vi "Shooter Button SUBVI.vi"   [LabVIEW 2011]
types:
  T1 = cluster{"Digital Input [1-16][0]":bool, "Digital Input [1-16][1]":bool, "Digital Input [1-16][2]":bool, "Digital Input [1-16][3]":bool, "Digital Input [1-16][4]":bool, "Digital Input [1-16][5]":bool, "Digital Input [1-16][6]":bool, "Digital Input [1-16][7]":bool, "Digital Input [1-16][8]":bool, "Digital Input [1-16][9]":bool, "Digital Input [1-16][10]":bool, "Digital Input [1-16][11]":bool, "Digital Input [1-16][12]":bool, "Digital Input [1-16][13]":bool, "Digital Input [1-16][14]":bool, "Digital Input [1-16][15]":bool}
  T2 = typedef "WPI_JoystickDevRef.ctl" = cluster{"Device":T3}
  T3 = typedef "WPI_JoystickDeviceEnum.ctl" = enum16{"USB 1", "USB 2", "USB 3", "USB 4", "Kinect 1", "Kinect 2"}
  T4 = typedef "WPI_JoystickButtonState.ctl" = cluster{"Button 1":bool, "Button 2":bool, "Button 3":bool, "Button 4":bool, "Button 5":bool, "Button 6":bool, "Button 7":bool, "Button 8":bool, "Button 9":bool, "Button 10":bool, "Button 11":bool, "Button 12":bool}
  T5 = cluster{"axis 1 (x)":dbl, "axis 2 (y)":dbl, "axis 3 (throttle)":dbl, "axis 4":dbl, "axis 5":dbl, "axis 6":dbl}
  T6 = typedef "WPI_DigitalInputDevRef.ctl" = cluster{"DevStatus":errorcluster, "DIO Channel":T7, "Digital Module":T8}
  T7 = typedef "FPGA_DIOChannel.ctl" = enum8{"DIO 1", "DIO 2", "DIO 3", "DIO 4", "DIO 5", "DIO 6", "DIO 7", "DIO 8", "DIO 9", "DIO 10", "DIO 11", "DIO 12", "DIO 13", "DIO 14", "Invalid"}
  T8 = typedef "FPGA_TypedefDigitalModule.ctl" = enum16{"Digital Module 1", "Digital Module 2"}
  T9 = typedef "WPI_MotorControlDeviceRef.ctl" = cluster{"DeviceStatus":errorcluster, "Type":enum16{"PWM", "CAN"}, "PWM":cluster{"Digital Module":T8, "PWM Channel":T10, "DeadBand":T11}, "CAN":cluster{"Device Number":u8, "Control Mode":T12, "Semaphore":T13, "Max Vout":dbl}, "Invert":bool, "TransformRef":T14, "InvTransformRef":T14}
  T10 = typedef "FPGA_DIOPWMChannel.ctl" = enum8{"PWM 1", "PWM 2", "PWM 3", "PWM 4", "PWM 5", "PWM 6", "PWM 7", "PWM 8", "PWM 9", "PWM 10", "Invalid"}
  T11 = typedef "WPI_PWMDeadband.ctl" = cluster{"Name":string, "maxPositivePwm":i32, "minPositivePwm":i32, "centerPwm":i32, "maxNegativePwm":i32, "minNegativePwm":i32, "angularRange":u16}
  T12 = typedef "WPI_CANJaguar_ControlMode.ctl" = enum8{"Percent VBus", "Current", "Speed", "Position", "Voltage"}
  T13 = typedef "Semaphore RefNum" = refnum<k1>
  T14 = typedef "WPI_PWMTransform_ConPane.ctl" = refnum<vi>
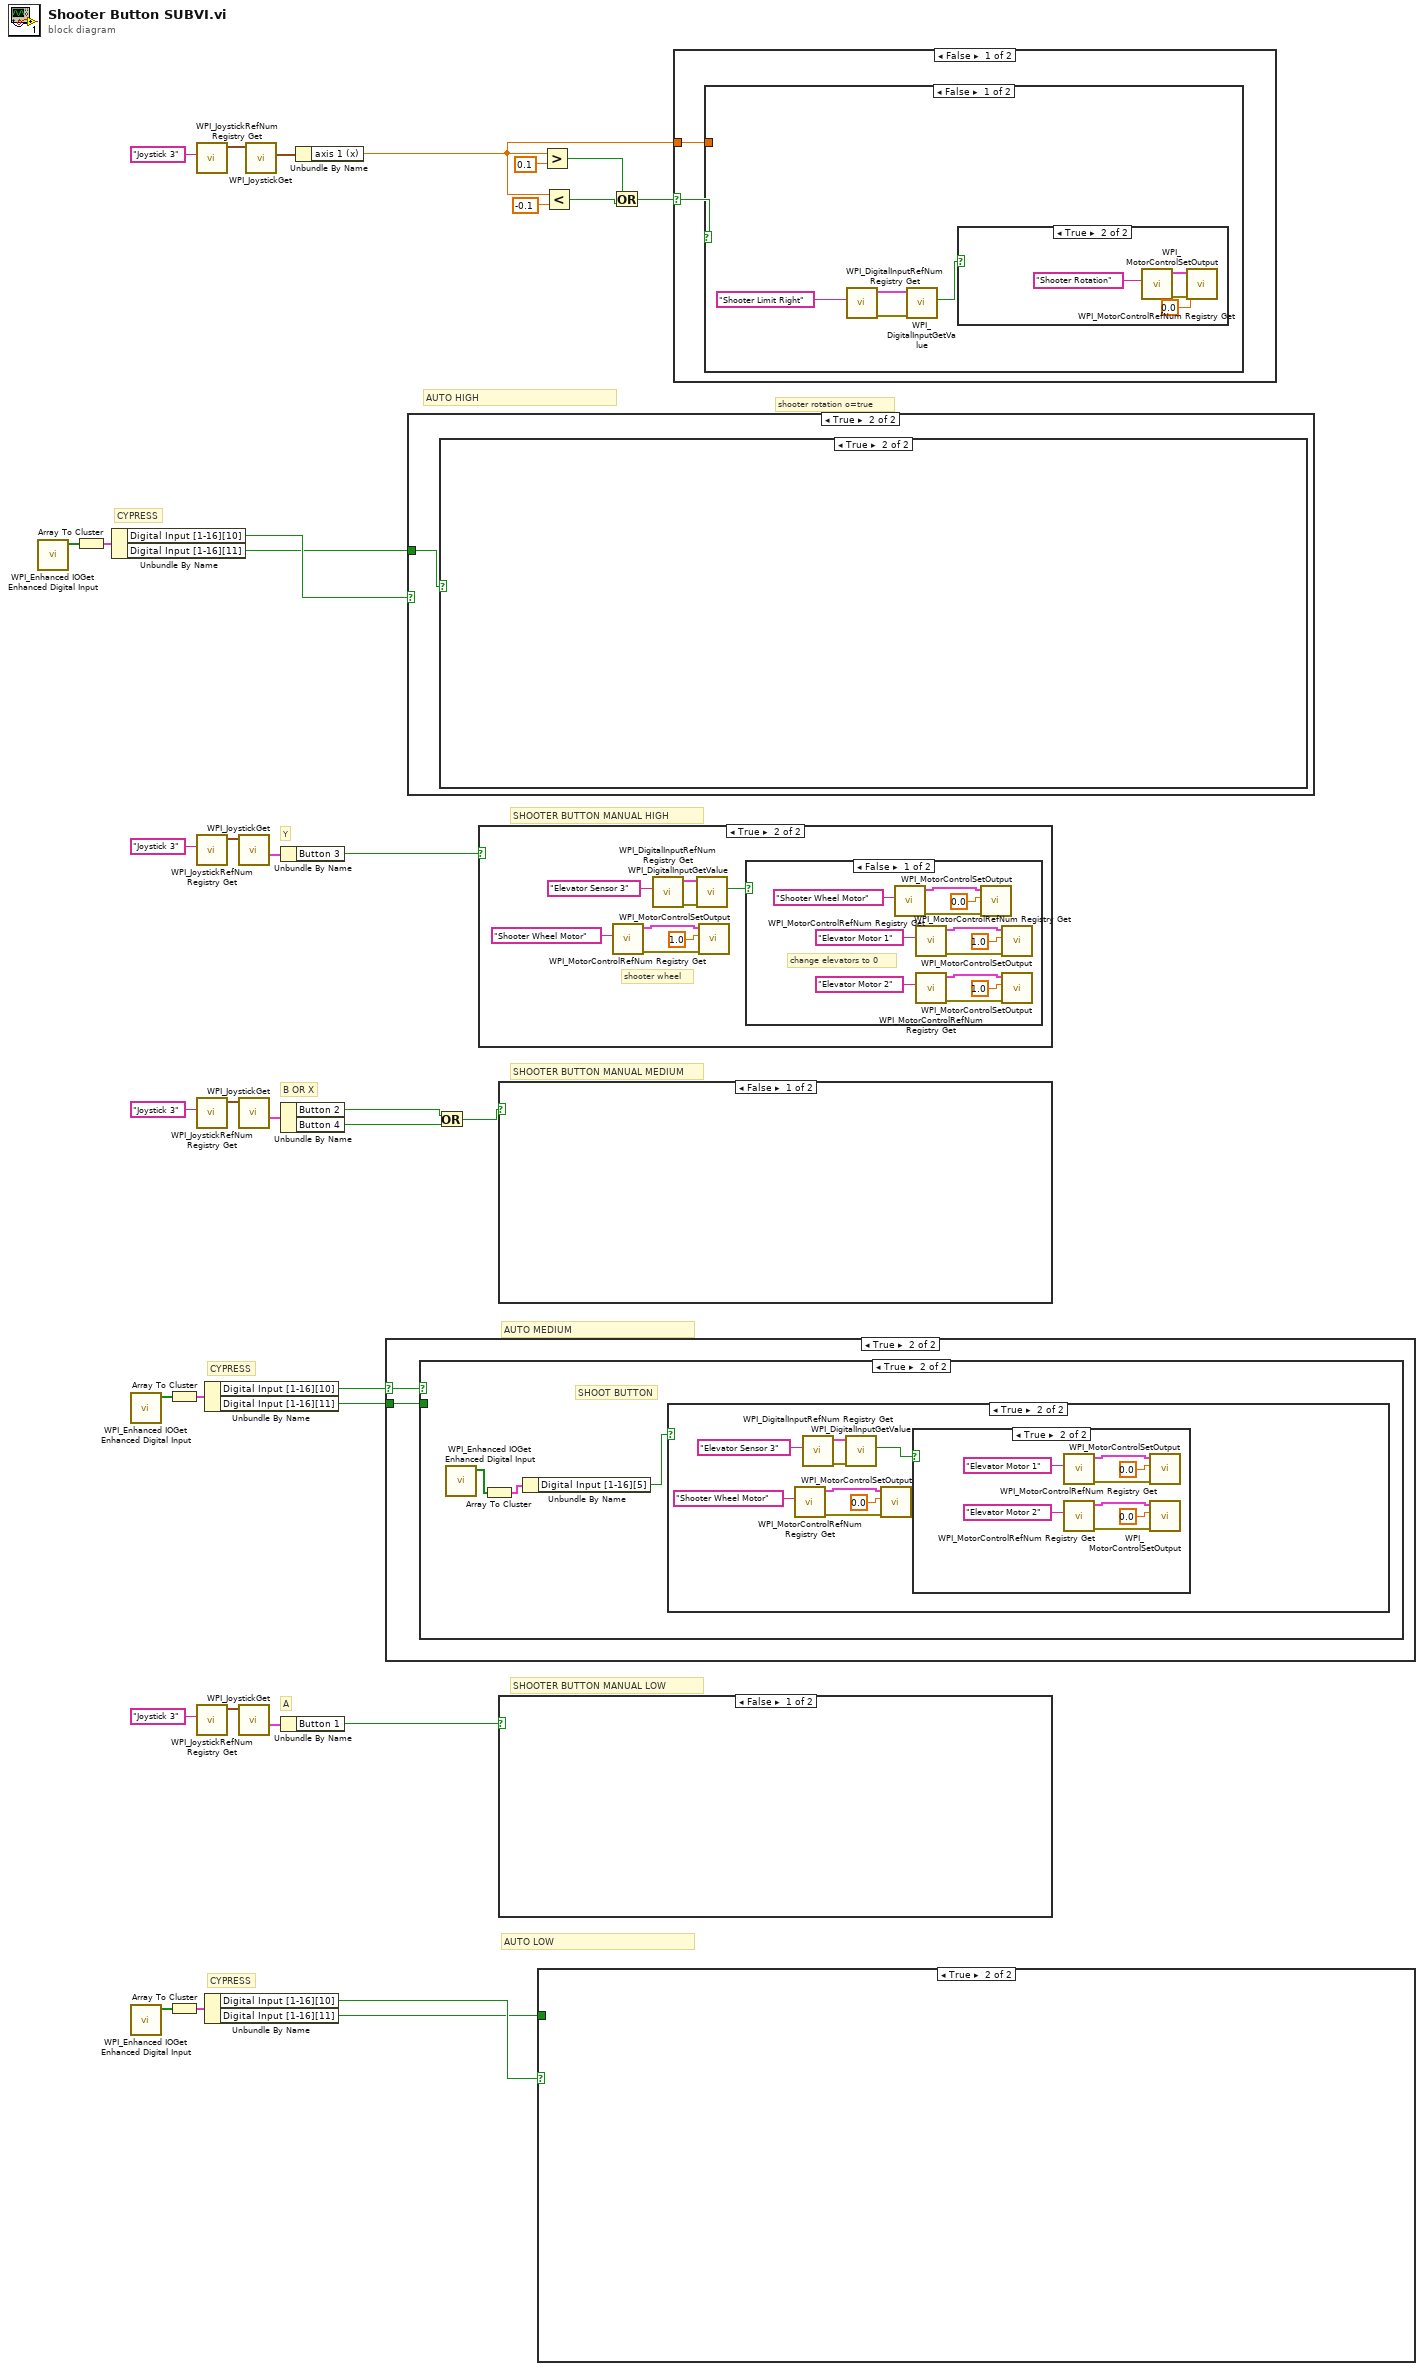
[diagram p0: block diagram]
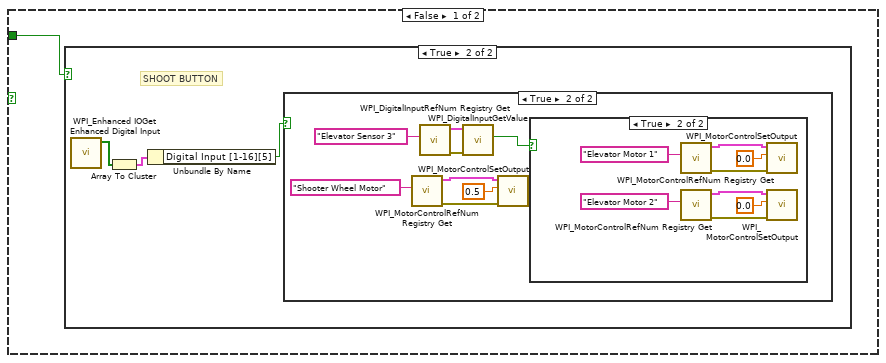
[diagram p2: hidden frame]
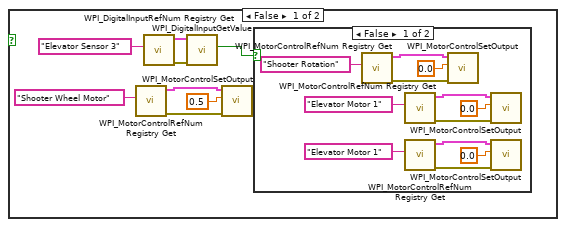
[diagram p4: hidden frame]
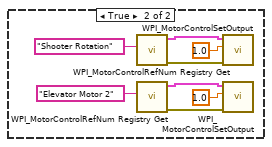
[diagram p5: hidden frame]
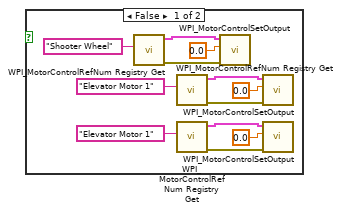
[diagram p6: hidden frame]
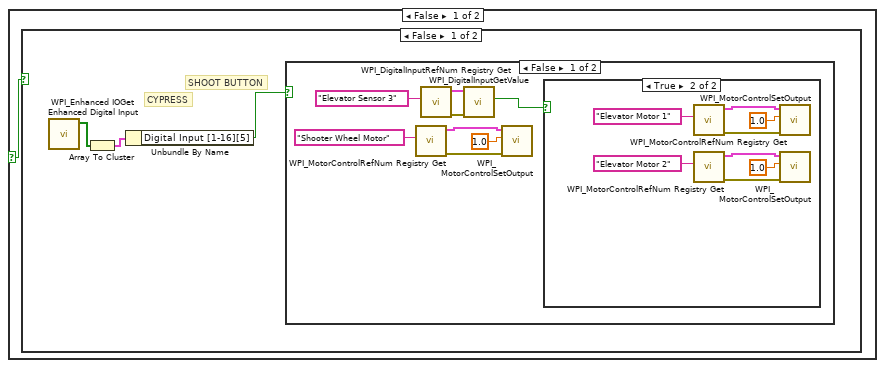
[diagram p8: hidden frame]
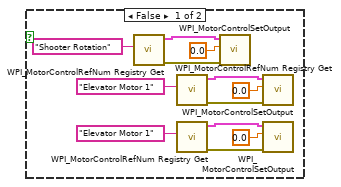
[diagram p9: hidden frame]
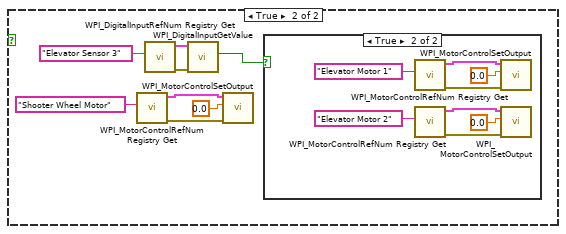
[diagram p10: hidden frame]
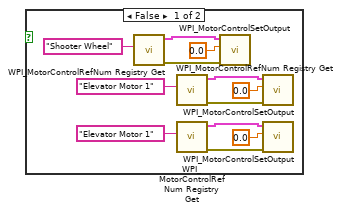
[diagram p11: hidden frame]
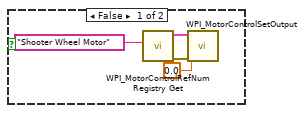
[diagram p13: hidden frame]
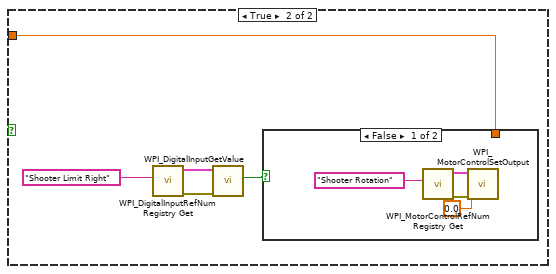
[diagram p14: hidden frame]
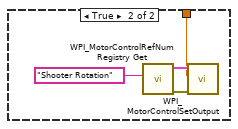
[diagram p15: hidden frame]
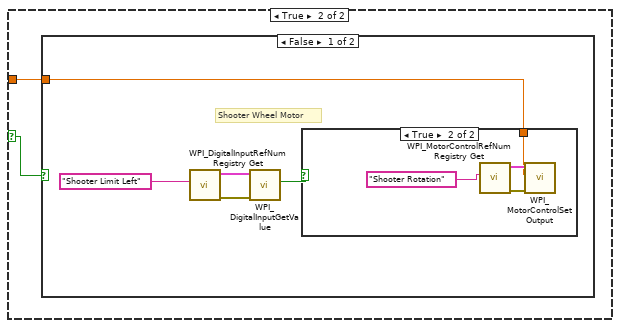
[diagram p16: hidden frame]
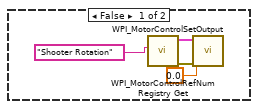
[diagram p17: hidden frame]
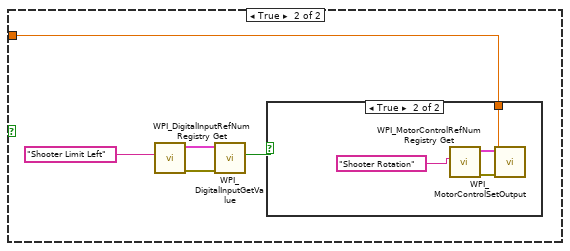
[diagram p18: hidden frame]
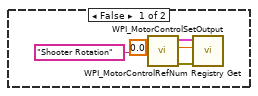
[diagram p19: hidden frame]
diagram:
  # "shooter rotation o=true"
  # "CYPRESS"
  # "CYPRESS"
  # "AUTO LOW"
  # "AUTO MEDIUM"
  # "A"
  # "B OR X"
  # "Y"
  # "SHOOTER BUTTON MANUAL LOW"
  # "SHOOTER BUTTON MANUAL MEDIUM"
  # "SHOOTER BUTTON MANUAL HIGH"
  # "CYPRESS"
  # "AUTO HIGH"
  n1 = call <vilib>:"WPI_Enhanced IOGet Enhanced Digital Input.vi"() -> ("Digital Input [1-16]"=w24:bool[])  [unwired: 10 in, 1 out]
  n2 = Array To Cluster(array=w24) -> (cluster=w23:T1)
  n3 = Unbundle By Name(w23) -> ("Digital Input [1-16][10]"=w8:bool, "Digital Input [1-16][11]"=w7:bool)
  n4 = call <vilib>:"WPI_Enhanced IOGet Enhanced Digital Input.vi"() -> ("Digital Input [1-16]"=w22:bool[])  [unwired: 10 in, 1 out]
  n5 = call <vilib>:"WPI_Enhanced IOGet Enhanced Digital Input.vi"() -> ("Digital Input [1-16]"=w20:bool[])  [unwired: 10 in, 1 out]
  n6 = Array To Cluster(array=w22) -> (cluster=w21:T1)
  n7 = Array To Cluster(array=w20) -> (cluster=w19:T1)
  n8 = call <vilib>:"WPI_JoystickRefNum Registry Get.vi"("refnum name"="Joystick 3") -> ("JoystickDevRef"=w17:T2)  [unwired: 9 in, 1 out]
  n9 = call <vilib>:"WPI_JoystickRefNum Registry Get.vi"("refnum name"="Joystick 3") -> ("JoystickDevRef"=w35:T2)  [unwired: 9 in, 1 out]
  n10 = call <vilib>:"WPI_JoystickRefNum Registry Get.vi"("refnum name"="Joystick 3") -> ("JoystickDevRef"=w32:T2)  [unwired: 9 in, 1 out]
  n11 = call <vilib>:"WPI_JoystickRefNum Registry Get.vi"("refnum name"="Joystick 3") -> ("JoystickDevRef"=w29:T2)  [unwired: 9 in, 1 out]
  n12 = Unbundle By Name(w21) -> ("Digital Input [1-16][10]"=w18:bool, "Digital Input [1-16][11]"=w6:bool)
  n13 = Unbundle By Name(w19) -> ("Digital Input [1-16][10]"=w5:bool, "Digital Input [1-16][11]"=w4:bool)
  n14 = call <vilib>:"WPI_JoystickGet.vi"("JoystickDevRef"=w35) -> ("Buttons"=w34:T4)  [unwired: 4 in, 2 out]
  n15 = call <vilib>:"WPI_JoystickGet.vi"("JoystickDevRef"=w32) -> ("Buttons"=w30:T4)  [unwired: 4 in, 2 out]
  n16 = call <vilib>:"WPI_JoystickGet.vi"("JoystickDevRef"=w29) -> ("Buttons"=w27:T4)  [unwired: 4 in, 2 out]
  n17 = call <vilib>:"WPI_JoystickGet.vi"("JoystickDevRef"=w17) -> ("Axes"=w15:T5)  [unwired: 4 in, 2 out]
  n18 = Unbundle By Name(w34) -> ("Button 3"=w33:bool)
  n19 = Unbundle By Name(w30) -> ("Button 2"=w3:bool, "Button 4"=w2:bool)
  n20 = Unbundle By Name(w27) -> ("Button 1"=w26:bool)
  n21 = Unbundle By Name(w15) -> ("axis 1 (x)"=w11:dbl)
  n22 = case shown="True" w18 {
    selector: w18 -> [_ w37]
    tunnel: w6 -> [_ w36]
    frame False {
    }
    frame True {
      n23 = case shown="True" w37 {
        tunnel: w36 -> [_ _]
        frame False {
        }
        frame True {
          # "SHOOT BUTTON"
          n24 = call <vilib>:"WPI_Enhanced IOGet Enhanced Digital Input.vi"() -> ("Digital Input [1-16]"=w40:bool[])  [unwired: 10 in, 1 out]
          n25 = Array To Cluster(array=w40) -> (cluster=w39:T1)
          n26 = Unbundle By Name(w39) -> ("Digital Input [1-16][5]"=w38:bool)
          n27 = case shown="True" w38 {
            frame False {
              n28 = call <vilib>:"WPI_DigitalInputRefNum Registry Get.vi"("refnum name"="Elevator Sensor 3") -> ("error out"=w47:errorcluster, "DigitalInputDevRef"=w46:T6)  [unwired: 9 in]
              n29 = call <vilib>:"WPI_MotorControlRefNum Registry Get.vi"("refnum name"="Shooter Wheel Motor") -> ("error out"=w44:errorcluster, "MotorControlDevRef"=w43:T9)  [unwired: 9 in]
              n30 = call <vilib>:"WPI_DigitalInputGetValue.vi"("error in (no error)"=w47, "DigitalInputDevRef"=w46) -> ("Value"=w45:bool)  [unwired: 7 in, 2 out]
              n31 = call <vilib>:"WPI_MotorControlSetOutput.vi"("error in (no error)"=w44, "Output"=0.75, "MotorControlDevRef"=w43) -> ()  [unwired: 7 in, 2 out]
              n32 = case shown="True" w45 {
                frame False {
                  n33 = call <vilib>:"WPI_MotorControlRefNum Registry Get.vi"("refnum name"="Shooter Rotation") -> ("error out"=w52:errorcluster, "MotorControlDevRef"=w51:T9)  [unwired: 9 in]
                  n34 = call <vilib>:"WPI_MotorControlRefNum Registry Get.vi"("refnum name"="Elevator Motor 1") -> ("error out"=w56:errorcluster, "MotorControlDevRef"=w55:T9)  [unwired: 9 in]
                  n35 = call <vilib>:"WPI_MotorControlRefNum Registry Get.vi"("refnum name"="Elevator Motor 1") -> ("error out"=w60:errorcluster, "MotorControlDevRef"=w59:T9)  [unwired: 9 in]
                  n36 = call <vilib>:"WPI_MotorControlSetOutput.vi"("error in (no error)"=w52, "Output"=0.0, "MotorControlDevRef"=w51) -> ()  [unwired: 7 in, 2 out]
                  n37 = call <vilib>:"WPI_MotorControlSetOutput.vi"("error in (no error)"=w56, "Output"=0.0, "MotorControlDevRef"=w55) -> ()  [unwired: 7 in, 2 out]
                  n38 = call <vilib>:"WPI_MotorControlSetOutput.vi"("error in (no error)"=w60, "Output"=0.0, "MotorControlDevRef"=w59) -> ()  [unwired: 7 in, 2 out]
                }
                frame True {
                  n39 = call <vilib>:"WPI_MotorControlRefNum Registry Get.vi"("refnum name"="Elevator Motor 1") -> ("error out"=w64:errorcluster, "MotorControlDevRef"=w63:T9)  [unwired: 9 in]
                  n40 = call <vilib>:"WPI_MotorControlRefNum Registry Get.vi"("refnum name"="Elevator Motor 2") -> ("error out"=w68:errorcluster, "MotorControlDevRef"=w67:T9)  [unwired: 9 in]
                  n41 = call <vilib>:"WPI_MotorControlSetOutput.vi"("error in (no error)"=w64, "Output"=1.0, "MotorControlDevRef"=w63) -> ()  [unwired: 7 in, 2 out]
                  n42 = call <vilib>:"WPI_MotorControlSetOutput.vi"("error in (no error)"=w68, "Output"=1.0, "MotorControlDevRef"=w67) -> ()  [unwired: 7 in, 2 out]
                }
              }
            }
            frame True {
              n43 = call <vilib>:"WPI_MotorControlRefNum Registry Get.vi"("refnum name"="Shooter Wheel Motor") -> ("error out"=w72:errorcluster, "MotorControlDevRef"=w71:T9)  [unwired: 9 in]
              n44 = call <vilib>:"WPI_DigitalInputRefNum Registry Get.vi"("refnum name"="Elevator Sensor 3") -> ("error out"=w75:errorcluster, "DigitalInputDevRef"=w74:T6)  [unwired: 9 in]
              n45 = call <vilib>:"WPI_DigitalInputGetValue.vi"("error in (no error)"=w75, "DigitalInputDevRef"=w74) -> ("Value"=w73:bool)  [unwired: 7 in, 2 out]
              n46 = call <vilib>:"WPI_MotorControlSetOutput.vi"("error in (no error)"=w72, "Output"=0.0, "MotorControlDevRef"=w71) -> ()  [unwired: 7 in, 2 out]
              n47 = case shown="True" w73 {
                frame False {
                  n48 = call <vilib>:"WPI_MotorControlRefNum Registry Get.vi"("refnum name"="Shooter Wheel") -> ("error out"=w80:errorcluster, "MotorControlDevRef"=w79:T9)  [unwired: 9 in]
                  n49 = call <vilib>:"WPI_MotorControlRefNum Registry Get.vi"("refnum name"="Elevator Motor 1") -> ("error out"=w84:errorcluster, "MotorControlDevRef"=w83:T9)  [unwired: 9 in]
                  n50 = call <vilib>:"WPI_MotorControlRefNum Registry Get.vi"("refnum name"="Elevator Motor 1") -> ("error out"=w88:errorcluster, "MotorControlDevRef"=w87:T9)  [unwired: 9 in]
                  n51 = call <vilib>:"WPI_MotorControlSetOutput.vi"("error in (no error)"=w80, "Output"=0.0, "MotorControlDevRef"=w79) -> ()  [unwired: 7 in, 2 out]
                  n52 = call <vilib>:"WPI_MotorControlSetOutput.vi"("error in (no error)"=w84, "Output"=0.0, "MotorControlDevRef"=w83) -> ()  [unwired: 7 in, 2 out]
                  n53 = call <vilib>:"WPI_MotorControlSetOutput.vi"("error in (no error)"=w88, "Output"=0.0, "MotorControlDevRef"=w87) -> ()  [unwired: 7 in, 2 out]
                }
                frame True {
                  n54 = call <vilib>:"WPI_MotorControlRefNum Registry Get.vi"("refnum name"="Elevator Motor 1") -> ("error out"=w92:errorcluster, "MotorControlDevRef"=w91:T9)  [unwired: 9 in]
                  n55 = call <vilib>:"WPI_MotorControlRefNum Registry Get.vi"("refnum name"="Elevator Motor 2") -> ("error out"=w96:errorcluster, "MotorControlDevRef"=w95:T9)  [unwired: 9 in]
                  n56 = call <vilib>:"WPI_MotorControlSetOutput.vi"("error in (no error)"=w92, "Output"=0.0, "MotorControlDevRef"=w91) -> ()  [unwired: 7 in, 2 out]
                  n57 = call <vilib>:"WPI_MotorControlSetOutput.vi"("error in (no error)"=w96, "Output"=0.0, "MotorControlDevRef"=w95) -> ()  [unwired: 7 in, 2 out]
                }
              }
            }
          }
        }
      }
    }
  }
  n58 = case shown="True" w8 {
    tunnel: w7 -> [_ w97]
    frame False {
    }
    frame True {
      n59 = case shown="True" w97 {
        selector: w97 -> [w98 _]
        frame False {
          n60 = case shown="False" w98 {
            frame False {
              # "CYPRESS"
              # "SHOOT BUTTON"
              n61 = call <vilib>:"WPI_Enhanced IOGet Enhanced Digital Input.vi"() -> ("Digital Input [1-16]"=w101:bool[])  [unwired: 10 in, 1 out]
              n62 = Array To Cluster(array=w101) -> (cluster=w100:T1)
              n63 = Unbundle By Name(w100) -> ("Digital Input [1-16][5]"=w99:bool)
              n64 = case shown="False" w99 {
                frame False {
                  n65 = call <vilib>:"WPI_MotorControlRefNum Registry Get.vi"("refnum name"="Shooter Wheel Motor") -> ("error out"=w105:errorcluster, "MotorControlDevRef"=w104:T9)  [unwired: 9 in]
                  n66 = call <vilib>:"WPI_DigitalInputRefNum Registry Get.vi"("refnum name"="Elevator Sensor 3") -> ("error out"=w108:errorcluster, "DigitalInputDevRef"=w107:T6)  [unwired: 9 in]
                  n67 = call <vilib>:"WPI_DigitalInputGetValue.vi"("error in (no error)"=w108, "DigitalInputDevRef"=w107) -> ("Value"=w106:bool)  [unwired: 7 in, 2 out]
                  n68 = call <vilib>:"WPI_MotorControlSetOutput.vi"("error in (no error)"=w105, "Output"=1.0, "MotorControlDevRef"=w104) -> ()  [unwired: 7 in, 2 out]
                  n69 = case shown="True" w106 {
                    frame False {
                      n70 = call <vilib>:"WPI_MotorControlRefNum Registry Get.vi"("refnum name"="Shooter Rotation") -> ("error out"=w113:errorcluster, "MotorControlDevRef"=w112:T9)  [unwired: 9 in]
                      n71 = call <vilib>:"WPI_MotorControlRefNum Registry Get.vi"("refnum name"="Elevator Motor 1") -> ("error out"=w117:errorcluster, "MotorControlDevRef"=w116:T9)  [unwired: 9 in]
                      n72 = call <vilib>:"WPI_MotorControlRefNum Registry Get.vi"("refnum name"="Elevator Motor 1") -> ("error out"=w121:errorcluster, "MotorControlDevRef"=w120:T9)  [unwired: 9 in]
                      n73 = call <vilib>:"WPI_MotorControlSetOutput.vi"("error in (no error)"=w113, "Output"=0.0, "MotorControlDevRef"=w112) -> ()  [unwired: 7 in, 2 out]
                      n74 = call <vilib>:"WPI_MotorControlSetOutput.vi"("error in (no error)"=w117, "Output"=0.0, "MotorControlDevRef"=w116) -> ()  [unwired: 7 in, 2 out]
                      n75 = call <vilib>:"WPI_MotorControlSetOutput.vi"("error in (no error)"=w121, "Output"=0.0, "MotorControlDevRef"=w120) -> ()  [unwired: 7 in, 2 out]
                    }
                    frame True {
                      n76 = call <vilib>:"WPI_MotorControlRefNum Registry Get.vi"("refnum name"="Elevator Motor 1") -> ("error out"=w125:errorcluster, "MotorControlDevRef"=w124:T9)  [unwired: 9 in]
                      n77 = call <vilib>:"WPI_MotorControlRefNum Registry Get.vi"("refnum name"="Elevator Motor 2") -> ("error out"=w129:errorcluster, "MotorControlDevRef"=w128:T9)  [unwired: 9 in]
                      n78 = call <vilib>:"WPI_MotorControlSetOutput.vi"("error in (no error)"=w125, "Output"=1.0, "MotorControlDevRef"=w124) -> ()  [unwired: 7 in, 2 out]
                      n79 = call <vilib>:"WPI_MotorControlSetOutput.vi"("error in (no error)"=w129, "Output"=1.0, "MotorControlDevRef"=w128) -> ()  [unwired: 7 in, 2 out]
                    }
                  }
                }
                frame True {
                  n80 = call <vilib>:"WPI_MotorControlRefNum Registry Get.vi"("refnum name"="Shooter Wheel Motor") -> ("error out"=w133:errorcluster, "MotorControlDevRef"=w132:T9)  [unwired: 9 in]
                  n81 = call <vilib>:"WPI_DigitalInputRefNum Registry Get.vi"("refnum name"="Elevator Sensor 3") -> ("error out"=w136:errorcluster, "DigitalInputDevRef"=w135:T6)  [unwired: 9 in]
                  n82 = call <vilib>:"WPI_DigitalInputGetValue.vi"("error in (no error)"=w136, "DigitalInputDevRef"=w135) -> ("Value"=w134:bool)  [unwired: 7 in, 2 out]
                  n83 = call <vilib>:"WPI_MotorControlSetOutput.vi"("error in (no error)"=w133, "Output"=0.0, "MotorControlDevRef"=w132) -> ()  [unwired: 7 in, 2 out]
                  n84 = case shown="True" w134 {
                    frame False {
                      n85 = call <vilib>:"WPI_MotorControlRefNum Registry Get.vi"("refnum name"="Shooter Wheel") -> ("error out"=w141:errorcluster, "MotorControlDevRef"=w140:T9)  [unwired: 9 in]
                      n86 = call <vilib>:"WPI_MotorControlRefNum Registry Get.vi"("refnum name"="Elevator Motor 1") -> ("error out"=w145:errorcluster, "MotorControlDevRef"=w144:T9)  [unwired: 9 in]
                      n87 = call <vilib>:"WPI_MotorControlRefNum Registry Get.vi"("refnum name"="Elevator Motor 1") -> ("error out"=w149:errorcluster, "MotorControlDevRef"=w148:T9)  [unwired: 9 in]
                      n88 = call <vilib>:"WPI_MotorControlSetOutput.vi"("error in (no error)"=w141, "Output"=0.0, "MotorControlDevRef"=w140) -> ()  [unwired: 7 in, 2 out]
                      n89 = call <vilib>:"WPI_MotorControlSetOutput.vi"("error in (no error)"=w145, "Output"=0.0, "MotorControlDevRef"=w144) -> ()  [unwired: 7 in, 2 out]
                      n90 = call <vilib>:"WPI_MotorControlSetOutput.vi"("error in (no error)"=w149, "Output"=0.0, "MotorControlDevRef"=w148) -> ()  [unwired: 7 in, 2 out]
                    }
                    frame True {
                      n91 = call <vilib>:"WPI_MotorControlRefNum Registry Get.vi"("refnum name"="Elevator Motor 1") -> ("error out"=w153:errorcluster, "MotorControlDevRef"=w152:T9)  [unwired: 9 in]
                      n92 = call <vilib>:"WPI_MotorControlRefNum Registry Get.vi"("refnum name"="Elevator Motor 2") -> ("error out"=w157:errorcluster, "MotorControlDevRef"=w156:T9)  [unwired: 9 in]
                      n93 = call <vilib>:"WPI_MotorControlSetOutput.vi"("error in (no error)"=w153, "Output"=0.0, "MotorControlDevRef"=w152) -> ()  [unwired: 7 in, 2 out]
                      n94 = call <vilib>:"WPI_MotorControlSetOutput.vi"("error in (no error)"=w157, "Output"=0.0, "MotorControlDevRef"=w156) -> ()  [unwired: 7 in, 2 out]
                    }
                  }
                }
              }
            }
            frame True {
            }
          }
        }
        frame True {
        }
      }
    }
  }
  n95 = Or(x=w3, y=w2) -> (x .or. y?=w1:bool)
  n96 = case shown="True" w33 {
    frame False {
    }
    frame True {
      # "shooter wheel"
      n97 = call <vilib>:"WPI_MotorControlRefNum Registry Get.vi"("refnum name"="Shooter Wheel Motor") -> ("error out"=w161:errorcluster, "MotorControlDevRef"=w160:T9)  [unwired: 9 in]
      n98 = call <vilib>:"WPI_DigitalInputRefNum Registry Get.vi"("refnum name"="Elevator Sensor 3") -> ("error out"=w164:errorcluster, "DigitalInputDevRef"=w163:T6)  [unwired: 9 in]
      n99 = call <vilib>:"WPI_DigitalInputGetValue.vi"("error in (no error)"=w164, "DigitalInputDevRef"=w163) -> ("Value"=w162:bool)  [unwired: 7 in, 2 out]
      n100 = call <vilib>:"WPI_MotorControlSetOutput.vi"("error in (no error)"=w161, "Output"=1.0, "MotorControlDevRef"=w160) -> ()  [unwired: 7 in, 2 out]
      n101 = case shown="False" w162 {
        frame False {
          # "change elevators to 0"
          n102 = call <vilib>:"WPI_MotorControlRefNum Registry Get.vi"("refnum name"="Shooter Wheel Motor") -> ("error out"=w169:errorcluster, "MotorControlDevRef"=w168:T9)  [unwired: 9 in]
          n103 = call <vilib>:"WPI_MotorControlRefNum Registry Get.vi"("refnum name"="Elevator Motor 1") -> ("error out"=w173:errorcluster, "MotorControlDevRef"=w172:T9)  [unwired: 9 in]
          n104 = call <vilib>:"WPI_MotorControlRefNum Registry Get.vi"("refnum name"="Elevator Motor 2") -> ("error out"=w177:errorcluster, "MotorControlDevRef"=w176:T9)  [unwired: 9 in]
          n105 = call <vilib>:"WPI_MotorControlSetOutput.vi"("error in (no error)"=w169, "Output"=0.0, "MotorControlDevRef"=w168) -> ()  [unwired: 7 in, 2 out]
          n106 = call <vilib>:"WPI_MotorControlSetOutput.vi"("error in (no error)"=w173, "Output"=1.0, "MotorControlDevRef"=w172) -> ()  [unwired: 7 in, 2 out]
          n107 = call <vilib>:"WPI_MotorControlSetOutput.vi"("error in (no error)"=w177, "Output"=1.0, "MotorControlDevRef"=w176) -> ()  [unwired: 7 in, 2 out]
        }
        frame True {
          n108 = call <vilib>:"WPI_MotorControlRefNum Registry Get.vi"("refnum name"="Elevator Motor Right") -> ("error out"=w181:errorcluster, "MotorControlDevRef"=w180:T9)  [unwired: 9 in]
          n109 = call <vilib>:"WPI_MotorControlRefNum Registry Get.vi"("refnum name"="Elevator Motor Left") -> ("error out"=w185:errorcluster, "MotorControlDevRef"=w184:T9)  [unwired: 9 in]
          n110 = call <vilib>:"WPI_MotorControlSetOutput.vi"("error in (no error)"=w181, "Output"=1.0, "MotorControlDevRef"=w180) -> ()  [unwired: 7 in, 2 out]
          n111 = call <vilib>:"WPI_MotorControlSetOutput.vi"("error in (no error)"=w185, "Output"=1.0, "MotorControlDevRef"=w184) -> ()  [unwired: 7 in, 2 out]
        }
      }
    }
  }
  n112 = case shown="False" w1 {
    frame False {
    }
    frame True {
      n113 = call <vilib>:"WPI_MotorControlRefNum Registry Get.vi"("refnum name"="Shooter Wheel Motor") -> ("error out"=w189:errorcluster, "MotorControlDevRef"=w188:T9)  [unwired: 9 in]
      n114 = call <vilib>:"WPI_DigitalInputRefNum Registry Get.vi"("refnum name"="Elevator Sensor 3") -> ("error out"=w192:errorcluster, "DigitalInputDevRef"=w191:T6)  [unwired: 9 in]
      n115 = call <vilib>:"WPI_MotorControlSetOutput.vi"("error in (no error)"=w189, "Output"=0.75, "MotorControlDevRef"=w188) -> ()  [unwired: 7 in, 2 out]
      n116 = call <vilib>:"WPI_DigitalInputGetValue.vi"("error in (no error)"=w192, "DigitalInputDevRef"=w191) -> ("Value"=w190:bool)  [unwired: 7 in, 2 out]
      n117 = case shown="False" w190 {
        frame False {
          n118 = call <vilib>:"WPI_MotorControlRefNum Registry Get.vi"("refnum name"="Shooter Wheel Motor") -> ("error out"=w197:errorcluster, "MotorControlDevRef"=w196:T9)  [unwired: 9 in]
          n119 = call <vilib>:"WPI_MotorControlRefNum Registry Get.vi"("refnum name"="Elevator Motor Right") -> ("error out"=w201:errorcluster, "MotorControlDevRef"=w200:T9)  [unwired: 9 in]
          n120 = call <vilib>:"WPI_MotorControlRefNum Registry Get.vi"("refnum name"="Elevator Motor Left") -> ("error out"=w205:errorcluster, "MotorControlDevRef"=w204:T9)  [unwired: 9 in]
          n121 = call <vilib>:"WPI_MotorControlSetOutput.vi"("error in (no error)"=w197, "Output"=0.0, "MotorControlDevRef"=w196) -> ()  [unwired: 7 in, 2 out]
          n122 = call <vilib>:"WPI_MotorControlSetOutput.vi"("error in (no error)"=w201, "Output"=0.0, "MotorControlDevRef"=w200) -> ()  [unwired: 7 in, 2 out]
          n123 = call <vilib>:"WPI_MotorControlSetOutput.vi"("error in (no error)"=w205, "Output"=0.0, "MotorControlDevRef"=w204) -> ()  [unwired: 7 in, 2 out]
        }
        frame True {
          n124 = call <vilib>:"WPI_MotorControlRefNum Registry Get.vi"("refnum name"="Elevator Motor Right") -> ("error out"=w209:errorcluster, "MotorControlDevRef"=w208:T9)  [unwired: 9 in]
          n125 = call <vilib>:"WPI_MotorControlRefNum Registry Get.vi"("refnum name"="Elevator Motor Left") -> ("error out"=w213:errorcluster, "MotorControlDevRef"=w212:T9)  [unwired: 9 in]
          n126 = call <vilib>:"WPI_MotorControlSetOutput.vi"("error in (no error)"=w209, "Output"=1.0, "MotorControlDevRef"=w208) -> ()  [unwired: 7 in, 2 out]
          n127 = call <vilib>:"WPI_MotorControlSetOutput.vi"("error in (no error)"=w213, "Output"=1.0, "MotorControlDevRef"=w212) -> ()  [unwired: 7 in, 2 out]
        }
      }
    }
  }
  n128 = case shown="False" w26 {
    frame False {
    }
    frame True {
      n129 = call <vilib>:"WPI_MotorControlRefNum Registry Get.vi"("refnum name"="Shooter Wheel Motor") -> ("error out"=w217:errorcluster, "MotorControlDevRef"=w216:T9)  [unwired: 9 in]
      n130 = call <vilib>:"WPI_DigitalInputRefNum Registry Get.vi"("refnum name"="Elevator Sensor 3") -> ("error out"=w220:errorcluster, "DigitalInputDevRef"=w219:T6)  [unwired: 9 in]
      n131 = call <vilib>:"WPI_MotorControlSetOutput.vi"("error in (no error)"=w217, "Output"=0.5, "MotorControlDevRef"=w216) -> ()  [unwired: 7 in, 2 out]
      n132 = call <vilib>:"WPI_DigitalInputGetValue.vi"("error in (no error)"=w220, "DigitalInputDevRef"=w219) -> ("Value"=w218:bool)  [unwired: 7 in, 2 out]
      n133 = case shown="False" w218 {
        frame False {
          n134 = call <vilib>:"WPI_MotorControlRefNum Registry Get.vi"("refnum name"="Shooter Wheel Motor") -> ("error out"=w225:errorcluster, "MotorControlDevRef"=w224:T9)  [unwired: 9 in]
          n135 = call <vilib>:"WPI_MotorControlRefNum Registry Get.vi"("refnum name"="Elevator Motor Right") -> ("error out"=w229:errorcluster, "MotorControlDevRef"=w228:T9)  [unwired: 9 in]
          n136 = call <vilib>:"WPI_MotorControlRefNum Registry Get.vi"("refnum name"="Elevator Motor Left") -> ("error out"=w233:errorcluster, "MotorControlDevRef"=w232:T9)  [unwired: 9 in]
          n137 = call <vilib>:"WPI_MotorControlSetOutput.vi"("error in (no error)"=w225, "Output"=0.0, "MotorControlDevRef"=w224) -> ()  [unwired: 7 in, 2 out]
          n138 = call <vilib>:"WPI_MotorControlSetOutput.vi"("error in (no error)"=w229, "Output"=0.0, "MotorControlDevRef"=w228) -> ()  [unwired: 7 in, 2 out]
          n139 = call <vilib>:"WPI_MotorControlSetOutput.vi"("error in (no error)"=w233, "Output"=0.0, "MotorControlDevRef"=w232) -> ()  [unwired: 7 in, 2 out]
        }
        frame True {
          n140 = call <vilib>:"WPI_MotorControlRefNum Registry Get.vi"("refnum name"="Elevator Motor Right") -> ("error out"=w237:errorcluster, "MotorControlDevRef"=w236:T9)  [unwired: 9 in]
          n141 = call <vilib>:"WPI_MotorControlRefNum Registry Get.vi"("refnum name"="Elevator Motor Left") -> ("error out"=w241:errorcluster, "MotorControlDevRef"=w240:T9)  [unwired: 9 in]
          n142 = call <vilib>:"WPI_MotorControlSetOutput.vi"("error in (no error)"=w237, "Output"=1.0, "MotorControlDevRef"=w236) -> ()  [unwired: 7 in, 2 out]
          n143 = call <vilib>:"WPI_MotorControlSetOutput.vi"("error in (no error)"=w241, "Output"=1.0, "MotorControlDevRef"=w240) -> ()  [unwired: 7 in, 2 out]
        }
      }
    }
  }
  n144 = case shown="True" w5 {
    tunnel: w4 -> [w242 _]
    frame False {
      n145 = case shown="True" w242 {
        frame False {
        }
        frame True {
          # "SHOOT BUTTON"
          n146 = call <vilib>:"WPI_Enhanced IOGet Enhanced Digital Input.vi"() -> ("Digital Input [1-16]"=w245:bool[])  [unwired: 10 in, 1 out]
          n147 = Array To Cluster(array=w245) -> (cluster=w244:T1)
          n148 = Unbundle By Name(w244) -> ("Digital Input [1-16][5]"=w243:bool)
          n149 = case shown="True" w243 {
            frame False {
              n150 = call <vilib>:"WPI_MotorControlRefNum Registry Get.vi"("refnum name"="Shooter Wheel Motor") -> ("error out"=w249:errorcluster, "MotorControlDevRef"=w248:T9)  [unwired: 9 in]
              n151 = call <vilib>:"WPI_DigitalInputRefNum Registry Get.vi"("refnum name"="Elevator Sensor 3") -> ("error out"=w252:errorcluster, "DigitalInputDevRef"=w251:T6)  [unwired: 9 in]
              n152 = call <vilib>:"WPI_DigitalInputGetValue.vi"("error in (no error)"=w252, "DigitalInputDevRef"=w251) -> ("Value"=w250:bool)  [unwired: 7 in, 2 out]
              n153 = call <vilib>:"WPI_MotorControlSetOutput.vi"("error in (no error)"=w249, "Output"=0.5, "MotorControlDevRef"=w248) -> ()  [unwired: 7 in, 2 out]
              n154 = case shown="False" w250 {
                frame False {
                  n155 = call <vilib>:"WPI_MotorControlRefNum Registry Get.vi"("refnum name"="Shooter Rotation") -> ("error out"=w257:errorcluster, "MotorControlDevRef"=w256:T9)  [unwired: 9 in]
                  n156 = call <vilib>:"WPI_MotorControlRefNum Registry Get.vi"("refnum name"="Elevator Motor 1") -> ("error out"=w261:errorcluster, "MotorControlDevRef"=w260:T9)  [unwired: 9 in]
                  n157 = call <vilib>:"WPI_MotorControlRefNum Registry Get.vi"("refnum name"="Elevator Motor 1") -> ("error out"=w265:errorcluster, "MotorControlDevRef"=w264:T9)  [unwired: 9 in]
                  n158 = call <vilib>:"WPI_MotorControlSetOutput.vi"("error in (no error)"=w257, "Output"=0.0, "MotorControlDevRef"=w256) -> ()  [unwired: 7 in, 2 out]
                  n159 = call <vilib>:"WPI_MotorControlSetOutput.vi"("error in (no error)"=w261, "Output"=0.0, "MotorControlDevRef"=w260) -> ()  [unwired: 7 in, 2 out]
                  n160 = call <vilib>:"WPI_MotorControlSetOutput.vi"("error in (no error)"=w265, "Output"=0.0, "MotorControlDevRef"=w264) -> ()  [unwired: 7 in, 2 out]
                }
                frame True {
                  n161 = call <vilib>:"WPI_MotorControlRefNum Registry Get.vi"("refnum name"="Shooter Rotation") -> ("error out"=w269:errorcluster, "MotorControlDevRef"=w268:T9)  [unwired: 9 in]
                  n162 = call <vilib>:"WPI_MotorControlRefNum Registry Get.vi"("refnum name"="Elevator Motor 2") -> ("error out"=w273:errorcluster, "MotorControlDevRef"=w272:T9)  [unwired: 9 in]
                  n163 = call <vilib>:"WPI_MotorControlSetOutput.vi"("error in (no error)"=w269, "Output"=1.0, "MotorControlDevRef"=w268) -> ()  [unwired: 7 in, 2 out]
                  n164 = call <vilib>:"WPI_MotorControlSetOutput.vi"("error in (no error)"=w273, "Output"=1.0, "MotorControlDevRef"=w272) -> ()  [unwired: 7 in, 2 out]
                }
              }
            }
            frame True {
              n165 = call <vilib>:"WPI_MotorControlRefNum Registry Get.vi"("refnum name"="Shooter Wheel Motor") -> ("error out"=w277:errorcluster, "MotorControlDevRef"=w276:T9)  [unwired: 9 in]
              n166 = call <vilib>:"WPI_DigitalInputRefNum Registry Get.vi"("refnum name"="Elevator Sensor 3") -> ("error out"=w280:errorcluster, "DigitalInputDevRef"=w279:T6)  [unwired: 9 in]
              n167 = call <vilib>:"WPI_DigitalInputGetValue.vi"("error in (no error)"=w280, "DigitalInputDevRef"=w279) -> ("Value"=w278:bool)  [unwired: 7 in, 2 out]
              n168 = call <vilib>:"WPI_MotorControlSetOutput.vi"("error in (no error)"=w277, "Output"=0.5, "MotorControlDevRef"=w276) -> ()  [unwired: 7 in, 2 out]
              n169 = case shown="True" w278 {
                frame False {
                  n170 = call <vilib>:"WPI_MotorControlRefNum Registry Get.vi"("refnum name"="Shooter Wheel") -> ("error out"=w285:errorcluster, "MotorControlDevRef"=w284:T9)  [unwired: 9 in]
                  n171 = call <vilib>:"WPI_MotorControlRefNum Registry Get.vi"("refnum name"="Elevator Motor 1") -> ("error out"=w289:errorcluster, "MotorControlDevRef"=w288:T9)  [unwired: 9 in]
                  n172 = call <vilib>:"WPI_MotorControlRefNum Registry Get.vi"("refnum name"="Elevator Motor 1") -> ("error out"=w293:errorcluster, "MotorControlDevRef"=w292:T9)  [unwired: 9 in]
                  n173 = call <vilib>:"WPI_MotorControlSetOutput.vi"("error in (no error)"=w285, "Output"=0.0, "MotorControlDevRef"=w284) -> ()  [unwired: 7 in, 2 out]
                  n174 = call <vilib>:"WPI_MotorControlSetOutput.vi"("error in (no error)"=w289, "Output"=0.0, "MotorControlDevRef"=w288) -> ()  [unwired: 7 in, 2 out]
                  n175 = call <vilib>:"WPI_MotorControlSetOutput.vi"("error in (no error)"=w293, "Output"=0.0, "MotorControlDevRef"=w292) -> ()  [unwired: 7 in, 2 out]
                }
                frame True {
                  n176 = call <vilib>:"WPI_MotorControlRefNum Registry Get.vi"("refnum name"="Elevator Motor 1") -> ("error out"=w297:errorcluster, "MotorControlDevRef"=w296:T9)  [unwired: 9 in]
                  n177 = call <vilib>:"WPI_MotorControlRefNum Registry Get.vi"("refnum name"="Elevator Motor 2") -> ("error out"=w301:errorcluster, "MotorControlDevRef"=w300:T9)  [unwired: 9 in]
                  n178 = call <vilib>:"WPI_MotorControlSetOutput.vi"("error in (no error)"=w297, "Output"=0.0, "MotorControlDevRef"=w296) -> ()  [unwired: 7 in, 2 out]
                  n179 = call <vilib>:"WPI_MotorControlSetOutput.vi"("error in (no error)"=w301, "Output"=0.0, "MotorControlDevRef"=w300) -> ()  [unwired: 7 in, 2 out]
                }
              }
            }
          }
        }
      }
    }
    frame True {
    }
  }
  n180 = Greater?(x=w11, y=0.1) -> (0:w10:bool)
  n181 = Less?(x=w11, y=-0.1) -> (x < y?=w9:bool)
  n182 = Or(x=w10, y=w9) -> (x .or. y?=w13:bool)
  n183 = case shown="False" w13 {
    selector: w13 -> [w302 w329]
    tunnel: w11 -> [w303 w330]
    frame False {
      n184 = case shown="False" w302 {
        tunnel: w303 -> [_ w320]
        frame False {
          n185 = call <vilib>:"WPI_DigitalInputRefNum Registry Get.vi"("refnum name"="Shooter Limit Right") -> ("error out"=w306:errorcluster, "DigitalInputDevRef"=w305:T6)  [unwired: 9 in]
          n186 = call <vilib>:"WPI_DigitalInputGetValue.vi"("error in (no error)"=w306, "DigitalInputDevRef"=w305) -> ("Value"=w304:bool)  [unwired: 7 in, 2 out]
          n187 = case shown="True" w304 {
            frame False {
              n188 = call <vilib>:"WPI_MotorControlRefNum Registry Get.vi"("refnum name"="Shooter Wheel Motor") -> ("error out"=w311:errorcluster, "MotorControlDevRef"=w309:T9)  [unwired: 9 in]
              n189 = call <vilib>:"WPI_MotorControlSetOutput.vi"("error in (no error)"=w311, "Output"=0.0, "MotorControlDevRef"=w309) -> ()  [unwired: 7 in, 2 out]
            }
            frame True {
              n190 = call <vilib>:"WPI_MotorControlRefNum Registry Get.vi"("refnum name"="Shooter Rotation") -> ("error out"=w314:errorcluster, "MotorControlDevRef"=w315:T9)  [unwired: 9 in]
              n191 = call <vilib>:"WPI_MotorControlSetOutput.vi"("error in (no error)"=w314, "Output"=0.0, "MotorControlDevRef"=w315) -> ()  [unwired: 7 in, 2 out]
            }
          }
        }
        frame True {
          n192 = call <vilib>:"WPI_DigitalInputRefNum Registry Get.vi"("refnum name"="Shooter Limit Right") -> ("error out"=w318:errorcluster, "DigitalInputDevRef"=w317:T6)  [unwired: 9 in]
          n193 = call <vilib>:"WPI_DigitalInputGetValue.vi"("error in (no error)"=w318, "DigitalInputDevRef"=w317) -> ("Value"=w316:bool)  [unwired: 7 in, 2 out]
          n194 = case shown="False" w316 {
            tunnel: w320 -> [_ w325]
            frame False {
              n195 = call <vilib>:"WPI_MotorControlRefNum Registry Get.vi"("refnum name"="Shooter Rotation") -> ("error out"=w324:errorcluster, "MotorControlDevRef"=w322:T9)  [unwired: 9 in]
              n196 = call <vilib>:"WPI_MotorControlSetOutput.vi"("error in (no error)"=w324, "Output"=0.0, "MotorControlDevRef"=w322) -> ()  [unwired: 7 in, 2 out]
            }
            frame True {
              n197 = call <vilib>:"WPI_MotorControlRefNum Registry Get.vi"("refnum name"="Shooter Rotation") -> ("error out"=w327:errorcluster, "MotorControlDevRef"=w328:T9)  [unwired: 9 in]
              n198 = call <vilib>:"WPI_MotorControlSetOutput.vi"("error in (no error)"=w327, "Output"=w325, "MotorControlDevRef"=w328) -> ()  [unwired: 7 in, 2 out]
            }
          }
        }
      }
    }
    frame True {
      n199 = case shown="False" w329 {
        tunnel: w330 -> [w331 w344]
        frame False {
          # "Shooter Wheel Motor"
          n200 = call <vilib>:"WPI_DigitalInputRefNum Registry Get.vi"("refnum name"="Shooter Limit Left") -> ("error out"=w333:errorcluster, "DigitalInputDevRef"=w332:T6)  [unwired: 9 in]
          n201 = call <vilib>:"WPI_DigitalInputGetValue.vi"("error in (no error)"=w333, "DigitalInputDevRef"=w332) -> ("Value"=w335:bool)  [unwired: 7 in, 2 out]
          n202 = case shown="True" w335 {
            tunnel: w331 -> [_ w340]
            frame False {
              n203 = call <vilib>:"WPI_MotorControlRefNum Registry Get.vi"("refnum name"="Shooter Rotation") -> ("error out"=w338:errorcluster, "MotorControlDevRef"=w336:T9)  [unwired: 9 in]
              n204 = call <vilib>:"WPI_MotorControlSetOutput.vi"("error in (no error)"=w338, "Output"=0.0, "MotorControlDevRef"=w336) -> ()  [unwired: 7 in, 2 out]
            }
            frame True {
              n205 = call <vilib>:"WPI_MotorControlRefNum Registry Get.vi"("refnum name"="Shooter Rotation") -> ("error out"=w342:errorcluster, "MotorControlDevRef"=w341:T9)  [unwired: 9 in]
              n206 = call <vilib>:"WPI_MotorControlSetOutput.vi"("error in (no error)"=w342, "Output"=w340, "MotorControlDevRef"=w341) -> ()  [unwired: 7 in, 2 out]
            }
          }
        }
        frame True {
          n207 = call <vilib>:"WPI_DigitalInputRefNum Registry Get.vi"("refnum name"="Shooter Limit Left") -> ("error out"=w346:errorcluster, "DigitalInputDevRef"=w345:T6)  [unwired: 9 in]
          n208 = call <vilib>:"WPI_DigitalInputGetValue.vi"("error in (no error)"=w346, "DigitalInputDevRef"=w345) -> ("Value"=w348:bool)  [unwired: 7 in, 2 out]
          n209 = case shown="True" w348 {
            tunnel: w344 -> [_ w354]
            frame False {
              n210 = call <vilib>:"WPI_MotorControlRefNum Registry Get.vi"("refnum name"="Shooter Rotation") -> ("error out"=w350:errorcluster, "MotorControlDevRef"=w351:T9)  [unwired: 9 in]
              n211 = call <vilib>:"WPI_MotorControlSetOutput.vi"("error in (no error)"=w350, "Output"=0.0, "MotorControlDevRef"=w351) -> ()  [unwired: 7 in, 2 out]
            }
            frame True {
              n212 = call <vilib>:"WPI_MotorControlRefNum Registry Get.vi"("refnum name"="Shooter Rotation") -> ("error out"=w353:errorcluster, "MotorControlDevRef"=w355:T9)  [unwired: 9 in]
              n213 = call <vilib>:"WPI_MotorControlSetOutput.vi"("error in (no error)"=w353, "Output"=w354, "MotorControlDevRef"=w355) -> ()  [unwired: 7 in, 2 out]
            }
          }
        }
      }
    }
  }
